vi "Main Tclk.vi"() -> ()   [LabVIEW 2018] (continued)
            n6367 = call "Email alert.vi"("Email log file path"=w2036, "Send email"=w2039, "Machine ID"=w2042, "Mail server"=w2041, "Alarm message"=w2037, "Recipents"=w2040) -> ()  [unwired: 6 in]
            n6368 = case shown="True" w2035 {
              frame False {
              }
              frame True {
                n6369 = stacked-sequence {
                  frame #0 {
                    n6370 = Wait (ms)(milliseconds to wait=u32 500) -> ()  [unwired: 1 out]
                  }
                  frame #1 {
                    w2067 = FALSE ("3D image paused active bypass")
                    n6371 = local write "Send reheat start email"(w2067) -> ()
                    "Reheat warning armed" <- w2067
                  }
                }
              }
            }
          }
          frame #14 {
            n6372 = local read "Start Reheat"() -> (w2079:bool)
            n6373 = local read "Reheat warning armed"() -> (w2078:bool)
            n6374 = local read "Reheat completed"() -> (w2075:bool)
            n6375 = local read "Machine Type"() -> (w2068:u8)
            n6376 = case shown="2" w2068 {
              tunnel: [w2098 w2120] -> w2072
              tunnel: [w2092 w2117] -> w2069
              frame 0, Default {
                w2084 = "%5.1f" ("format string")
                w2086 = "%#g" ("format string")
                n6377 = local read "Reheat Output"() -> (w2106:T21)
                n6378 = local read "HV Data Output"() -> (w2093:T18)
                n6379 = Unbundle By Name(w2106) -> ("Initial emission (uA)"=w2105:sgl, "Initial suppressor (V)"=w2104:sgl, "V/I Slope"=w2097:sgl, "Reheat Success"=w2092:bool)
                n6380 = Unbundle By Name(w2093) -> ("Suppressor (V)"=w2091:sgl, "Emission (uA)"=w2089:sgl)
                n6381 = Format Into String(format string=w2084, w2105) -> (resulting string=w2102:string)  [unwired: 2 in, 1 out]
                n6382 = Format Into String(format string=w2084, w2097) -> (resulting string=w2096:string)  [unwired: 2 in, 1 out]
                n6383 = Format Into String(format string=w2086, w2091) -> (resulting string=w2090:string)  [unwired: 2 in, 1 out]
                n6384 = Format Into String(format string=w2086, w2104) -> (resulting string=w2100:string)  [unwired: 2 in, 1 out]
                n6385 = Format Into String(format string="%3.1f", w2089) -> (resulting string=w2088:string)  [unwired: 2 in, 1 out]
                n6386 = Concatenate Strings("FIB reheat completed successfully, initial emission: " ("Alarm message"), w2102, " uA @ suppressor = " ("element"), w2100, " V, V/I slope = " ("element"), w2096, ", suppressor = " ("string"), w2090, " V @ " ("string"), w2088, " uA emission " ("string")) -> (w2098:string)
              }
              frame 2 {
                w2107 = "%3.1f" ("format string")
                n6387 = local read "Capella HV Data Output"() -> (w2118:T17)
                n6388 = local read "Reheat Output"() -> (w2121:T21)
                n6389 = Unbundle By Name(w2121) -> ("Reheat Success"=w2117:bool)
                n6390 = Unbundle By Name(w2118) -> ("Suppressor (V)"=w2116:sgl, "Emission Actual (uA)"=w2114:sgl)
                n6391 = local read "FIB V/I slope"() -> (w2109:sgl)
                n6392 = Format Into String(format string=w2107, w2109) -> (resulting string=w2108:string)  [unwired: 2 in, 1 out]
                n6393 = Format Into String(format string="%5.1f", w2116) -> (resulting string=w2115:string)  [unwired: 2 in, 1 out]
                n6394 = Format Into String(format string=w2107, w2114) -> (resulting string=w2113:string)  [unwired: 2 in, 1 out]
                n6395 = Concatenate Strings("FIB reheat completed successfully, suppressor =  " ("Alarm message"), w2115, " V @ " ("string"), w2113, " uA emission, V/I slope =  " ("string"), w2108) -> (w2120:string)
              }
            }
            n6396 = local read "Mail server"() -> (w2081:string)
            n6397 = local read "Hardware Configuration"() -> (w2083:T25)
            n6398 = Not(x=w2079) -> (.not. x?=w2076:bool)
            n6399 = Not(x=w2078) -> (.not. x?=w2077:bool)
            n6400 = Unbundle By Name(w2083) -> ("Machine ID"=w2082:string)
            n6401 = Compound Arithmetic op=AND(w2076, w2077, w2075) -> (w2080:bool)
            n6402 = local read "Email Alert Recipients"() -> (w2071:string[])
            n6403 = local read "Email Log Files"() -> (w2070:path)
            n6404 = case shown="True" w2076 {
              frame False {
              }
              frame True {
                n6405 = stacked-sequence {
                  frame #0 {
                    n6406 = Wait (ms)(milliseconds to wait=u32 500) -> ()  [unwired: 1 out]
                  }
                  frame #1 {
                    n6407 = local write "Reheat warning armed"(TRUE ("3D image paused active bypass")) -> ()
                  }
                }
              }
            }
            n6408 = Select(t=w2072, s=w2069, f="FIB reheat failed" ("Alarm message")) -> (s? t:f=w2074:string)
            n6409 = call "Email alert.vi"("Email log file path"=w2070, "Send email"=w2080, "Machine ID"=w2082, "Mail server"=w2081, "Alarm message"=w2074, "Recipents"=w2071) -> ()  [unwired: 6 in]
          }
          frame #15 {
            n6410 = local read "Email Alert Recipients"() -> (w2129:string[])
            n6411 = local read "Auto re-engage"() -> (w2125:bool)
            n6412 = local read "Re-engage warning armed"() -> (w2126:bool)
            n6413 = local read "Mail server"() -> (w2130:string)
            n6414 = local read "Hardware Configuration"() -> (w2132:T25)
            n6415 = local read "Email Log Files"() -> (w2124:path)
            n6416 = Unbundle By Name(w2132) -> ("Machine ID"=w2131:string)
            n6417 = Compound Arithmetic op=AND(w2125, w2126) -> (w2127:bool)
            n6418 = call "Email alert.vi"("Email log file path"=w2124, "Send email"=w2127, "Machine ID"=w2131, "Mail server"=w2130, "Alarm message"="Auto re-engaging started", "Recipents"=w2129) -> ()  [unwired: 6 in]
            n6419 = case shown="True" w2125 {
              frame False {
              }
              frame True {
                n6420 = stacked-sequence {
                  frame #0 {
                    n6421 = Wait (ms)(milliseconds to wait=u32 500) -> ()  [unwired: 1 out]
                  }
                  frame #1 {
                    "Re-engage warning armed" <- FALSE ("3D image paused active bypass")
                  }
                }
              }
            }
          }
          frame #16 {
            n6422 = local read "Email Alert Recipients"() -> (w2148:string[])
            n6423 = local read "Auto re-engage"() -> (w2140:bool)
            n6424 = local read "Re-engage warning armed"() -> (w2144:bool)
            n6425 = local read "Re-engage cancelled"() -> (w2136:bool)
            n6426 = local read "Re-engage counts"() -> (w2138:u8)
            n6427 = local read "Mail server"() -> (w2149:string)
            n6428 = local read "Hardware Configuration"() -> (w2151:T25)
            n6429 = local read "Email Log Files"() -> (w2141:path)
            n6430 = Not Equal?(x=w2139, y=w2138) -> (x != y?=w2137:bool)
            n6431 = Equal?(x=w2138, y=u8 50) -> (x = y?=w2142:bool)
            n6432 = Unbundle By Name(w2151) -> ("Machine ID"=w2150:string)
            n6433 = Not(x=w2144) -> (.not. x?=w2145:bool)
            n6434 = Not(x=w2136) -> (.not. x?=w2135:bool)
            n6435 = Compound Arithmetic op=AND(w2140, w2145, w2135, w2137, w2142) -> (w2146:bool)
            n6436 = call "Email alert.vi"("Email log file path"=w2141, "Send email"=w2146, "Machine ID"=w2150, "Mail server"=w2149, "Alarm message"="FI has not covered after 50 frames", "Recipents"=w2148) -> ()  [unwired: 6 in]
            n6437 = case shown="True" w2140 {
              frame False {
              }
              frame True {
                n6438 = stacked-sequence {
                  frame #0 {
                    n6439 = Wait (ms)(milliseconds to wait=u32 500) -> ()  [unwired: 1 out]
                  }
                  frame #1 {
                  }
                }
              }
            }
          }
          frame #17 {
            n6440 = local read "Email Alert Recipients"() -> (w2166:string[])
            n6441 = local read "Auto re-engage"() -> (w2158:bool)
            n6442 = local read "Re-engage warning armed"() -> (w2162:bool)
            n6443 = local read "Re-engage cancelled"() -> (w2154:bool)
            n6444 = local read "Re-engage counts"() -> (w2157:u8)
            n6445 = local read "Mail server"() -> (w2167:string)
            n6446 = local read "Hardware Configuration"() -> (w2169:T25)
            n6447 = local read "Email Log Files"() -> (w2159:path)
            n6448 = Not Equal?(x=w2156, y=w2157) -> (x != y?=w2155:bool)
            n6449 = Equal?(x=w2157, y=u8 100) -> (x = y?=w2160:bool)
            n6450 = Unbundle By Name(w2169) -> ("Machine ID"=w2168:string)
            n6451 = Not(x=w2162) -> (.not. x?=w2163:bool)
            n6452 = Not(x=w2154) -> (.not. x?=w2153:bool)
            n6453 = Compound Arithmetic op=AND(w2158, w2163, w2153, w2155, w2160) -> (w2164:bool)
            n6454 = call "Email alert.vi"("Email log file path"=w2159, "Send email"=w2164, "Machine ID"=w2168, "Mail server"=w2167, "Alarm message"="FI has not covered after 100 frames", "Recipents"=w2166) -> ()  [unwired: 6 in]
            n6455 = case shown="True" w2158 {
              frame False {
              }
              frame True {
                n6456 = stacked-sequence {
                  frame #0 {
                    n6457 = Wait (ms)(milliseconds to wait=u32 500) -> ()  [unwired: 1 out]
                  }
                  frame #1 {
                  }
                }
              }
            }
          }
          frame #18 {
            n6458 = local read "Email Alert Recipients"() -> (w2184:string[])
            n6459 = local read "Auto re-engage"() -> (w2176:bool)
            n6460 = local read "Re-engage warning armed"() -> (w2180:bool)
            n6461 = local read "Re-engage cancelled"() -> (w2172:bool)
            n6462 = local read "Re-engage counts"() -> (w2175:u8)
            n6463 = local read "Mail server"() -> (w2185:string)
            n6464 = local read "Hardware Configuration"() -> (w2187:T25)
            n6465 = local read "Email Log Files"() -> (w2177:path)
            n6466 = Not Equal?(x=w2174, y=w2175) -> (x != y?=w2173:bool)
            n6467 = Equal?(x=w2175, y=u8 200) -> (x = y?=w2178:bool)
            n6468 = Unbundle By Name(w2187) -> ("Machine ID"=w2186:string)
            n6469 = Not(x=w2180) -> (.not. x?=w2181:bool)
            n6470 = Not(x=w2172) -> (.not. x?=w2171:bool)
            n6471 = Compound Arithmetic op=AND(w2176, w2181, w2171, w2173, w2178) -> (w2182:bool)
            n6472 = call "Email alert.vi"("Email log file path"=w2177, "Send email"=w2182, "Machine ID"=w2186, "Mail server"=w2185, "Alarm message"="FI has not covered after 200 frames", "Recipents"=w2184) -> ()  [unwired: 6 in]
            n6473 = case shown="True" w2176 {
              frame False {
              }
              frame True {
                n6474 = stacked-sequence {
                  frame #0 {
                    n6475 = Wait (ms)(milliseconds to wait=u32 500) -> ()  [unwired: 1 out]
                  }
                  frame #1 {
                  }
                }
              }
            }
          }
          frame #19 {
            n6476 = local read "Auto re-engage"() -> (w2202:bool)
            n6477 = local read "Re-engage warning armed"() -> (w2200:bool)
            n6478 = local read "Re-engage cancelled"() -> (w2190:bool)
            n6479 = local read "Email Alert Recipients"() -> (w2204:string[])
            n6480 = local read "Re-engage counts"() -> (w2194:u8)
            n6481 = local read "Mail server"() -> (w2205:string)
            n6482 = local read "Hardware Configuration"() -> (w2207:T25)
            n6483 = local read "Email Log Files"() -> (w2199:path)
            n6484 = Not(x=w2202) -> (.not. x?=w2201:bool)
            n6485 = Subtract(x=w2194, y=u8 12) -> (x-y=w2193:u8)
            n6486 = Unbundle By Name(w2207) -> ("Machine ID"=w2206:string)
            n6487 = Not(x=w2200) -> (.not. x?=w2191:bool)
            n6488 = Not(x=w2190) -> (.not. x?=w2189:bool)
            n6489 = Format Into String(w2193) -> (resulting string=w2196:string)  [unwired: 3 in, 1 out]
            n6490 = Compound Arithmetic op=AND(w2201, w2191, w2189) -> (w2203:bool)
            n6491 = Concatenate Strings("Auto re-engaging finished, FI recovered in " ("Alarm message"), w2196, " frames" ("Alarm message")) -> (w2197:string)
            n6492 = call "Email alert.vi"("Email log file path"=w2199, "Send email"=w2203, "Machine ID"=w2206, "Mail server"=w2205, "Alarm message"=w2197, "Recipents"=w2204) -> ()  [unwired: 6 in]
            n6493 = case shown="True" w2201 {
              frame False {
              }
              frame True {
                n6494 = stacked-sequence {
                  frame #0 {
                    n6495 = Wait (ms)(milliseconds to wait=u32 500) -> ()  [unwired: 1 out]
                  }
                  frame #1 {
                    n6496 = local write "Re-engage warning armed"(TRUE ("3D image paused active bypass")) -> ()
                  }
                }
              }
            }
          }
          frame #20 {
            n6497 = local read "Auto re-engage"() -> (w2218:bool)
            n6498 = local read "Re-engage cancelled"() -> (w2210:bool)
            n6499 = local read "Email Alert Recipients"() -> (w2220:string[])
            n6500 = local read "Re-engage counts"() -> (w2211:u8)
            n6501 = local read "Mail server"() -> (w2221:string)
            n6502 = local read "Hardware Configuration"() -> (w2223:T25)
            n6503 = local read "Email Log Files"() -> (w2216:path)
            n6504 = Not(x=w2218) -> (.not. x?=w2217:bool)
            n6505 = Unbundle By Name(w2223) -> ("Machine ID"=w2222:string)
            n6506 = Format Into String(w2211) -> (resulting string=w2213:string)  [unwired: 3 in, 1 out]
            n6507 = Compound Arithmetic op=AND(w2217, w2210) -> (w2219:bool)
            n6508 = Concatenate Strings("Auto re-engaging cancelled after " ("Alarm message"), w2213, " frames" ("Alarm message")) -> (w2214:string)
            n6509 = call "Email alert.vi"("Email log file path"=w2216, "Send email"=w2219, "Machine ID"=w2222, "Mail server"=w2221, "Alarm message"=w2214, "Recipents"=w2220) -> ()  [unwired: 6 in]
            n6510 = case shown="True" w2217 {
              frame False {
              }
              frame True {
                n6511 = stacked-sequence {
                  frame #0 {
                    n6512 = Wait (ms)(milliseconds to wait=u32 500) -> ()  [unwired: 1 out]
                  }
                  frame #1 {
                    "Re-engage cancelled" <- FALSE ("3D image paused active bypass")
                  }
                }
              }
            }
          }
          frame #21 {
            w2227 = "%5.3f" ("format string")
            n6513 = local read "FIB"() -> (w2226:bool)
            n6514 = local read "Focus index warning active"() -> (w2231:bool)
            n6515 = local read "Alert Settings"() -> (w2235:T36)
            n6516 = local read "Email Alert Recipients"() -> (w2243:string[])
            n6517 = local read "Focus Index"() -> (w2228:sgl)
            n6518 = local read "Mail server"() -> (w2244:string)
            n6519 = local read "Hardware Configuration"() -> (w2246:T25)
            n6520 = local read "Focus index warning armed"() -> (w2241:bool)
            n6521 = Unbundle By Name(w2235) -> ("Focus index warning"=w2232:bool, "Focus index low limit"=w2234:sgl, "Run Auto Stig"=w2233:bool)
            n6522 = Unbundle By Name(w2246) -> ("Machine ID"=w2245:string)
            n6523 = Format Into String(format string=w2227, w2234) -> (resulting string=w2237:string)  [unwired: 2 in, 1 out]
            n6524 = Compound Arithmetic op=AND(w2226, w2231, w2241, w2232) -> (w2242:bool)
            n6525 = Format Into String(format string=w2227, w2228) -> (resulting string=w2240:string)  [unwired: 2 in, 1 out]
            n6526 = local read "Email Log Files"() -> (w2229:path)
            n6527 = Compound Arithmetic op=AND(w2231, w2232, w2233) -> (w2230:bool)
            n6528 = Concatenate Strings("Focus index dropped below " ("Alarm message"), w2237, " to " ("Alarm message"), w2240) -> (w2239:string)
            n6529 = call "Email alert.vi"("Email log file path"=w2229, "Send email"=w2242, "Machine ID"=w2245, "Mail server"=w2244, "Alarm message"=w2239, "Recipents"=w2243) -> ()  [unwired: 6 in]
            n6530 = case shown="True" w2231 {
              frame False {
              }
              frame True {
                n6531 = stacked-sequence {
                  frame #0 {
                    n6532 = Wait (ms)(milliseconds to wait=u32 500) -> ()  [unwired: 1 out]
                  }
                  frame #1 {
                    "Focus index warning armed" <- FALSE ("3D image paused active bypass")
                  }
                }
              }
            }
            n6533 = case shown="True" w2230 {
              frame False {
              }
              frame True {
                n6534 = local write "Auto Stig"(TRUE ("Auto Stig")) -> ()
              }
            }
          }
          frame #22 {
            w2254 = "%5.3f" ("format string")
            n6535 = local read "Focus index stop trigger active"() -> (w2259:bool)
            n6536 = local read "Alert Settings"() -> (w2262:T36)
            n6537 = local read "Email Alert Recipients"() -> (w2268:string[])
            n6538 = local read "Focus Index"() -> (w2255:sgl)
            n6539 = local read "Z removal stop threshold Z(nm)"() -> (w2250:u8)
            n6540 = local read "Mail server"() -> (w2269:string)
            n6541 = local read "Hardware Configuration"() -> (w2271:T25)
            n6542 = Unbundle By Name(w2262) -> ("Focus index warning"=w2260:bool, "Focus index stop limit"=w2261:sgl)
            n6543 = Unbundle By Name(w2271) -> ("Machine ID"=w2270:string)
            n6544 = Format Into String(format string=w2254, w2261) -> (resulting string=w2264:string)  [unwired: 2 in, 1 out]
            n6545 = Format Into String(format string=w2254, w2255) -> (resulting string=w2267:string)  [unwired: 2 in, 1 out]
            n6546 = Format Into String(format string="%d", w2250) -> (resulting string=w2252:string)  [unwired: 2 in, 1 out]
            n6547 = Compound Arithmetic op=AND(w2259, w2260) -> (w2256:bool)
            n6548 = local read "Email Log Files"() -> (w2258:path)
            n6549 = Concatenate Strings("Focus index dropped below " ("Alarm message"), w2264, " to " ("Alarm message"), w2267, " for " ("string"), w2252, "nm removal" ("string")) -> (w2266:string)
            n6550 = call "Email alert.vi"("Email log file path"=w2258, "Send email"=w2256, "Machine ID"=w2270, "Mail server"=w2269, "Alarm message"=w2266, "Recipents"=w2268) -> ()  [unwired: 6 in]
            n6551 = case shown="True" w2256 {
              frame False {
              }
              frame True {
                n6552 = stacked-sequence {
                  frame #0 {
                    n6553 = Wait (ms)(milliseconds to wait=u32 500) -> ()  [unwired: 1 out]
                  }
                  frame #1 {
                    n6554 = local write "Focus index stop trigger active"(FALSE ("Focus index stop trigger active")) -> ()
                    n6555 = local write "FI below limit counts"(u8 0 ("FI below limit counts")) -> ()
                  }
                }
              }
            }
          }
          frame #23 {
            n6556 = local read "Email Alert Recipients"() -> (w2287:string[])
            n6557 = local read "Focus index recovery active"() -> (w2284:bool)
            n6558 = local read "Focus index warning armed"() -> (w2285:bool)
            n6559 = local read "Alert Settings"() -> (w2279:T36)
            n6560 = local read "Focus Index"() -> (w2276:sgl)
            n6561 = local read "Mail server"() -> (w2288:string)
            n6562 = local read "Hardware Configuration"() -> (w2290:T25)
            n6563 = Unbundle By Name(w2279) -> ("Focus index warning"=w2278:bool)
            n6564 = Not(x=w2285) -> (.not. x?=w2280:bool)
            n6565 = Unbundle By Name(w2290) -> ("Machine ID"=w2289:string)
            n6566 = Compound Arithmetic op=AND(w2284, w2280, w2278) -> (w2286:bool)
            n6567 = Format Into String(format string="%5.3f", w2276) -> (resulting string=w2283:string)  [unwired: 2 in, 1 out]
            n6568 = local read "Email Log Files"() -> (w2277:path)
            n6569 = Concatenate Strings("Focus index recovered to " ("Alarm message"), w2283) -> (w2282:string)
            n6570 = call "Email alert.vi"("Email log file path"=w2277, "Send email"=w2286, "Machine ID"=w2289, "Mail server"=w2288, "Alarm message"=w2282, "Recipents"=w2287) -> ()  [unwired: 6 in]
            n6571 = case shown="True" w2284 {
              frame False {
              }
              frame True {
                n6572 = stacked-sequence {
                  frame #0 {
                    n6573 = Wait (ms)(milliseconds to wait=u32 500) -> ()  [unwired: 1 out]
                  }
                  frame #1 {
                    n6574 = local write "Focus index warning armed"(TRUE ("Focus index warning armed")) -> ()
                  }
                }
              }
            }
          }
          frame #24 {
            w2294 = "%5.3f" ("format string")
            n6575 = local read "Temp (F)"() -> (w2305:sgl)
            n6576 = local read "Temp range (F)"() -> (w2300:sgl)
            n6577 = local read "Temp gradient (F/min)"() -> (w2304:dbl)
            n6578 = local read "Mail server"() -> (w2313:string)
            n6579 = local read "Hardware Configuration"() -> (w2315:T25)
            n6580 = local read "Alert Settings"() -> (w2297:T36)
            n6581 = Format Into String(format string=w2294, w2305) -> (resulting string=w2309:string)  [unwired: 2 in, 1 out]
            n6582 = Format Into String(format string=w2294, w2300) -> (resulting string=w2298:string)  [unwired: 2 in, 1 out]
            n6583 = local read "Email Alert Recipients"() -> (w2312:string[])
            n6584 = local read "FIB"() -> (w2293:bool)
            n6585 = local read "Temperature warning active"() -> (w2303:bool)
            n6586 = local read "Temperature warning armed"() -> (w2302:bool)
            n6587 = Unbundle By Name(w2315) -> ("Machine ID"=w2314:string)
            n6588 = Format Into String(format string=w2294, w2304) -> (resulting string=w2307:string)  [unwired: 2 in, 1 out]
            n6589 = Unbundle By Name(w2297) -> ("Temperature alarm"=w2296:bool)
            n6590 = Concatenate Strings("Temperature reached " ("Alarm message"), w2309, " F, range @ " ("Alarm message"), w2298, " F, gradient @ " ("Alarm message"), w2307, " F/min" ("string")) -> (w2310:string)
            n6591 = local read "Email Log Files"() -> (w2295:path)
            n6592 = Compound Arithmetic op=AND(w2293, w2303, w2302, w2296) -> (w2301:bool)
            n6593 = call "Email alert.vi"("Email log file path"=w2295, "Send email"=w2301, "Machine ID"=w2314, "Mail server"=w2313, "Alarm message"=w2310, "Recipents"=w2312) -> ()  [unwired: 6 in]
            n6594 = case shown="True" w2303 {
              frame False {
              }
              frame True {
                n6595 = stacked-sequence {
                  frame #0 {
                    n6596 = Wait (ms)(milliseconds to wait=u32 500) -> ()  [unwired: 1 out]
                  }
                  frame #1 {
                    "Temperature warning armed" <- FALSE ("3D image paused active bypass")
                  }
                }
              }
            }
          }
          frame #25 {
            w2319 = "%5.3f" ("format string")
            n6597 = local read "Temp (F)"() -> (w2329:sgl)
            n6598 = local read "Temp range (F)"() -> (w2326:sgl)
            n6599 = local read "Temp gradient (F/min)"() -> (w2328:dbl)
            n6600 = local read "Mail server"() -> (w2337:string)
            n6601 = local read "Hardware Configuration"() -> (w2339:T25)
            n6602 = local read "Email Alert Recipients"() -> (w2336:string[])
            n6603 = local read "Alert Settings"() -> (w2322:T36)
            n6604 = Format Into String(format string=w2319, w2329) -> (resulting string=w2333:string)  [unwired: 2 in, 1 out]
            n6605 = Format Into String(format string=w2319, w2326) -> (resulting string=w2324:string)  [unwired: 2 in, 1 out]
            n6606 = local read "FIB"() -> (w2318:bool)
            n6607 = local read "Temperature recovery active"() -> (w2323:bool)
            n6608 = local read "Temperature warning armed"() -> (w2340:bool)
            n6609 = Format Into String(format string=w2319, w2328) -> (resulting string=w2331:string)  [unwired: 2 in, 1 out]
            n6610 = Unbundle By Name(w2322) -> ("Temperature alarm"=w2321:bool)
            n6611 = Unbundle By Name(w2339) -> ("Machine ID"=w2338:string)
            n6612 = Concatenate Strings("Temperature recovered to " ("Alarm message"), w2333, " F, range @ " ("Alarm message"), w2324, " F, gradient @ " ("Alarm message"), w2331, " F/min" ("string")) -> (w2334:string)
            n6613 = Not(x=w2340) -> (.not. x?=w2341:bool)
            n6614 = local read "Email Log Files"() -> (w2320:path)
            n6615 = Compound Arithmetic op=AND(w2318, w2323, w2341, w2321) -> (w2327:bool)
            n6616 = call "Email alert.vi"("Email log file path"=w2320, "Send email"=w2327, "Machine ID"=w2338, "Mail server"=w2337, "Alarm message"=w2334, "Recipents"=w2336) -> ()  [unwired: 6 in]
            n6617 = case shown="True" w2323 {
              frame False {
              }
              frame True {
                n6618 = stacked-sequence {
                  frame #0 {
                    n6619 = Wait (ms)(milliseconds to wait=u32 500) -> ()  [unwired: 1 out]
                  }
                  frame #1 {
                    n6620 = local write "Temperature warning armed"(TRUE ("Focus index warning armed")) -> ()
                  }
                }
              }
            }
          }
        }
        n6621 = Wait Until Next ms Multiple(millisecond multiple=u32 1000) -> ()  [unwired: 1 out]
        n6622 = local read "Stop"() -> (w1831:bool)
      }
      n6623 = Unregister For Events(event registration refnum=w713, error in=w714) -> (error out=w711:errorcluster)
      n6624 = Close Reference(reference=w715, error in (no error)=w711) -> ()  [unwired: 1 out]
      n6625 = while {
        stop <- w1208 stop-if-true
        n6626 = Wait Until Next ms Multiple(millisecond multiple=u32 100) -> ()  [unwired: 1 out]
        n6627 = case shown="True" "Load recipe" {
          frame False {
          }
          frame True {
            n6628 = stacked-sequence {
              frame #0 {
                n6629 = call "Recipe read write.vi"("Write"=FALSE, "Recipe path"="Read recipe path") -> ("Read output"=w1211:T114)  [unwired: 6 in, 3 out]
                n6630 = local read "Milling para"() -> (w1225:T35)
                n6631 = local read "FIB"() -> (w1236:bool)
                n6632 = Unbundle By Name(w1211) -> ("SEM Scan Parameters"=w1226:T5, "Detector Information"=w1227:T8, "SEM Options"=w1228:T27, "Focus Index Options"=w1210:T28, "Image fit to"=w1215:u8, "File Information"=w1229:T31, "Low mag SEM"=w1230:T30, "Mid Mag SEM"=w1219:T115, "FIB-SEM Angle"=w1231:dbl, "Milling para"=w1232:T35, "FI Detector"=w1237:u16, "Auto Optimzation"=w1238:bool, "Images per Auto Optimization"=w1239:u16, "AF Range (nm)"=w1240:sgl, "AF Steps"=w1241:u8, "AS Range (%)"=w1242:sgl, "AS Steps"=w1243:u8, "AA Range (%)"=w1217:sgl, "AA Steps"=w1216:u8, "X shift (nm/frame)"=w1234:dbl, "Y shift (nm/frame)"=w1233:dbl, "FIB Y zoom pixel (nm)"=w1235:dbl, "Mail server"=w1244:string, "Email Alert Recipients"=w1245:string[], "Alert Settings"=w1218:T116, "Reheat Parameters"=w1214:T1, "Start FIB HV DataLog"=w1213:bool, "Interval (s)"=w1212:u16)
                n6633 = local write "Recipe input"(w1211) -> ()
                n6634 = Not(x=w1236) -> (.not. x?=w1223:bool)
                n6635 = Unbundle By Name(w1225) -> ("Mill start from Last"=w1224:bool)
                n6636 = local write "Focus Index Options"(w1210) -> ()
                n6637 = local write "Image fit to"(w1215) -> ()
                n6638 = local write "FI Detector"(w1237) -> ()
                n6639 = local write "Auto Optimzation"(w1238) -> ()
                n6640 = local write "Images per Auto Optimization"(w1239) -> ()
                n6641 = local write "AF Range (nm)"(w1240) -> ()
                n6642 = local write "AF Steps"(w1241) -> ()
                n6643 = local write "AS Range (%)"(w1242) -> ()
                n6644 = local write "AS Steps"(w1243) -> ()
                n6645 = local write "AA Range (%)"(w1217) -> ()
                n6646 = local write "AA Steps"(w1216) -> ()
                n6647 = local write "Alert Settings"(w1218) -> ()
                n6648 = local write "Reheat Parameters"(w1214) -> ()
                n6649 = local write "Start FIB HV DataLog"(w1213) -> ()
                n6650 = local write "Interval (s)"(w1212) -> ()
                n6651 = Or(x=w1224, y=w1223) -> (x .or. y?=w1222:bool)
                n6652 = case shown="True" w1222 {
                  tunnel: w1226 -> [w1249 w1306]
                  tunnel: w1227 -> [_ w1292]
                  tunnel: w1228 -> [_ w1305]
                  tunnel: w1229 -> [_ w1304]
                  tunnel: w1230 -> [w1248 w1303]
                  tunnel: w1231 -> [_ w1302]
                  tunnel: w1232 -> [w1247 w1301]
                  tunnel: w1233 -> [_ w1300]
                  tunnel: w1234 -> [_ w1299]
                  tunnel: w1235 -> [_ w1298]
                  tunnel: w1244 -> [_ w1297]
                  tunnel: w1245 -> [_ w1296]
                  tunnel: w1219 -> [w1246 w1295]
                  frame False {
                    n6653 = stacked-sequence {
                      tunnel: w1249 -> [w1260 _ _]
                      tunnel: w1248 -> [_ w1280 _]
                      tunnel: w1247 -> [_ _ w1286]
                      tunnel: w1246 -> [_ w1272 _]
                      frame #0 {
                        n6654 = Unbundle By Name(w1260) -> ("X size (um)"=w1259:sgl, "Y size (um)"=w1258:sgl, "X size (V)"=w1257:dbl, "X size auto"=w1256:bool, "Scan rate (Hz)"=w1255:u32, "Oversampling"=w1254:u32, "Oversampling auto"=w1253:bool, "Frame line rampdown ratio"=w1252:sgl, "Pixel size (nm)"=w1251:sgl)
                        n6655 = local read "SEM Scan Parameters"() -> (w1261:T26)
                        n6656 = Bundle By Name(cluster=w1261, "X size (um)"=w1259, "Y size (um)"=w1258, "X size (V)"=w1257, "X size auto"=w1256, "Scan rate (Hz)"=w1255, "Oversampling"=w1254, "Oversampling auto"=w1253, "Frame line rampdown ratio"=w1252, "Pixel size (nm)"=w1251) -> (w1250:T26)
                        n6657 = local write "SEM Scan Parameters"(w1250) -> ()
                      }
                      frame #1 {
                        n6658 = Unbundle By Name(w1280) -> ("Low mag scan"=w1277:bool, "Prior to main scan"=w1276:bool, "Low mag interval"=w1275:u32, "Low mag scan rate (Hz)"=w1274:u32, "Show HM box"=w1273:bool)
                        n6659 = Unbundle By Name(w1272) -> ("Mid mag scan"=w1269:bool, "Prior to main scan"=w1268:bool, "Mid mag interval"=w1267:u32, "X size (um)"=w1266:sgl, "Y size (um)"=w1265:sgl, "Mid mag scan rate (Hz)"=w1264:u32, "Pixel size (nm)"=w1263:dbl, "Show MM box"=w1262:bool)
                        n6660 = local read "Mid Mag SEM"() -> (w1270:T29)
                        n6661 = Bundle By Name(cluster=w1270, "Mid mag scan"=w1269, "Prior to main scan"=w1268, "Mid mag interval"=w1267, "X size (um)"=w1266, "Y size (um)"=w1265, "Mid mag scan rate (Hz)"=w1264, "Pixel size (nm)"=w1263, "Show MM box"=w1262) -> (w1271:T29)
                        n6662 = local read "Low Mag SEM"() -> (w1279:T30)
                        n6663 = Bundle By Name(cluster=w1279, "Low mag scan"=w1277, "Prior to main scan"=w1276, "Low mag interval"=w1275, "Low mag scan rate (Hz)"=w1274, "Show HM box"=w1273) -> (w1278:T30)
                        n6664 = local write "Low Mag SEM"(w1278) -> ()
                        n6665 = local write "Mid Mag SEM"(w1271) -> ()
                      }
                      frame #2 {
                        n6666 = Unbundle By Name(w1286) -> ("Line milling time (s)"=w1283:sgl, "Lines auto pause"=w1282:u16, "Auto Profile"=w1281:bool)
                        n6667 = local read "Milling para"() -> (w1285:T35)
                        n6668 = Bundle By Name(cluster=w1285, "Line milling time (s)"=w1283, "Lines auto pause"=w1282, "Auto Profile"=w1281) -> (w1284:T35)
                        n6669 = local write "Milling para"(w1284) -> ()
                      }
                    }
                  }
                  frame True {
                    n6670 = local write "SEM Scan Parameters"(w1306) -> ()
                    n6671 = local write "Detector Information"(w1292) -> ()
                    n6672 = local write "SEM Options"(w1305) -> ()
                    n6673 = local write "File Information"(w1304) -> ()
                    n6674 = local write "Low Mag SEM"(w1303) -> ()
                    n6675 = local write "Mid Mag SEM"(w1295) -> ()
                    n6676 = local write "FIB-SEM Angle"(w1302) -> ()
                    n6677 = local write "Milling para"(w1301) -> ()
                    n6678 = local write "X shift (nm/image)"(w1299) -> ()
                    n6679 = local write "Y shift (nm/image)"(w1300) -> ()
                    n6680 = local write "FIB Y zoom pixel (nm)"(w1298) -> ()
                    n6681 = local write "Mail server"(w1297) -> ()
                    n6682 = local write "Email Alert Recipients"(w1296) -> ()
                    n6683 = Unbundle By Name(w1292) -> ("Brightness A"=w1291:dbl, "Contrast A"=w1290:dbl, "Detector B name"=w1289:string, "Brightness B"=w1288:dbl, "Contrast B"=w1287:dbl)
                    n6684 = local read "Hardware Configuration"() -> (w1294:T25)
                    n6685 = Bundle By Name(cluster=w1294, "Brightness A"=w1291, "Contrast A"=w1290, "Detector B name"=w1289, "Brightness B"=w1288, "Contrast B"=w1287) -> (w1293:T25)
                    n6686 = local write "Hardware Configuration"(w1293) -> ()
                  }
                }
              }
              frame #1 {
                n6687 = local read "Milling para"() -> (w1329:T35)
                n6688 = local read "FIB"() -> (w1328:bool)
                n6689 = case shown="False" w1328 {
                  tunnel: [TRUE ("Origin") FALSE ("Origin")] -> w1327
                  tunnel: [0.0 ("Y offset pre (um)") w1332] -> w1309
                  frame False {
                  }
                  frame True {
                    n6690 = local read "Y offset pre (um)"() -> (w1332:dbl)
                  }
                }
                n6691 = Unbundle By Name(w1329) -> ("X size (um)"=w1316:sgl, "Z size (um)"=w1317:sgl, "Z-step (nm)"=w1307:dbl)
                n6692 = expression code="x/1e3"(w1307) -> (w1319:dbl)
                n6693 = control-ref of="FIB Image"() -> (w1323:refnum<vi>)
                n6694 = local read "FIB Scan Parameters"() -> (w1324:T32)
                n6695 = local read "FIB Options"() -> (w1325:T33)
                n6696 = shared-variable ".\\Zeiss Library.lvlib\\Milling Z Voltage RT"() -> (w1326:sgl)  [unwired: 1 in, 1 out]
                n6697 = expression code="log2( x/0.1)"(w1316) -> (w1314:sgl)
                n6698 = Round Toward +Infinity(x=w1314) -> (ceil(x): smallest int >= x=w1312:sgl)
                n6699 = call "FIB image draw milling.vi"("Milling Z Voltage"=w1326, "Milling para"=w1329, "Z offset pre (um)"=w1309, "FIB Options"=w1325, "FIB Scan Parameters"=w1324, "Origin"=w1327, "Image reference"=w1323) -> ("Trapezoidal"=w1308:cluster{"X":i16, "Y":i16}[])  [unwired: 3 in, 1 out]
                n6700 = Scale By Power Of 2(n=w1312, x=ext 1.0) -> (x*2^n=w1315:ext)
                n6701 = local write "Trapezoidal"(w1308) -> ()
                n6702 = Divide(x=w1317, y=w1319) -> (x/y=w1311:dbl)
                n6703 = Round To Nearest(number=w1311) -> (nearest integer value=w1322:dbl)
                n6704 = local read "Milling para"() -> (w1320:T35)
                n6705 = Increment(x=w1322) -> (x+1=w1321:dbl)
                n6706 = Multiply(x=w1322, y=w1319) -> (x*y=w1318:dbl)
                n6707 = Bundle By Name(cluster=w1320, "X resolution"=w1315, "Z resolution"=w1321, "Z size (um)"=w1318) -> (w1310:T35)
                n6708 = local write "Milling para"(w1310) -> ()
              }
              frame #2 {
                n6709 = local read "dat to csv and xml"() -> (w1334:bool)
                n6710 = local write "Load recipe"(FALSE ("Load recipe")) -> ()
                n6711 = case shown="True" w1334 {
                  frame False {
                  }
                  frame True {
                    n6712 = stacked-sequence {
                      frame #0 {
                        w1350 = i16 60 ("top")
                        n6713 = local read "SEM Scan Parameters"() -> (w1345:T26)
                        n6714 = local read "Recipe input"() -> (w1378:T7)
                        n6715 = local read "Last FIB recipe"() -> (w1379:path)
                        n6716 = local read "Read recipe path"() -> (w1364:path)
                        n6717 = Path To String(path=w1364) -> (string=w1363:string)
                        n6718 = call "Recipe read write.vi"("Write"=TRUE, "Recipe path"=w1379, "Write input"=w1378) -> ()  [unwired: 5 in, 4 out]
                        n6719 = call "Zeiss File Header Tclk.vi"("Write"=FALSE, "Input file path"=w1364) -> ("Ouputs"=w1373:T79)  [unwired: 7 in, 2 out]
                        n6720 = Unbundle By Name(w1345) -> ("X size (um)"=w1344:sgl, "Y size (um)"=w1341:sgl, "Pixel size (nm)"=w1343:sgl)
                        n6721 = local read "Hardware Configuration"() -> (w1337:T25)
                        n6722 = Unbundle By Name(w1373) -> ("Data Logging.Milling Z voltage (V)"=w1371:sgl, "Data Logging.FIB slice #"=w1369:u32, "Data Logging.Focus Index"=w1368:sgl, "Decimating factor"=w1338:u16)
                        n6723 = call "Timestamp from dat file.vi"("dat file path"=w1364) -> ("time stamp"=w1370:timestamp)  [unwired: 10 in]
                        n6724 = Search and Replace String(input string=w1363, search string=".dat", replace string=".png" ("replace string (\"\")")) -> (result string=w1360:string)  [unwired: 5 in, 3 out]
                        n6725 = String To Path(string=w1360) -> (path=w1359:path)
                        n6726 = local read "Last milling snapshot"() -> (w1374:path)
                        n6727 = expression code="x/1000"(w1343) -> (w1342:sgl)
                        n6728 = Divide(x=w1344, y=w1342) -> (x/y=w1340:sgl)
                        n6729 = Divide(x=w1341, y=w1342) -> (x/y=w1339:sgl)
                        n6730 = Unbundle By Name(w1337) -> ("SEM Max FOV (um)"=w1336:sgl)
                        n6731 = Divide(x=w1340, y=w1338) -> (x/y=w1352:sgl)
                        n6732 = Divide(x=w1339, y=w1338) -> (x/y=w1349:sgl)
                        n6733 = To Word Integer(number=w1352) -> (16bit integer=w1348:i16)
                        n6734 = To Word Integer(number=w1349) -> (16bit integer=w1347:i16)
                        n6735 = local read "Re-engage Files"() -> (w1354:path)
                        n6736 = Bundle(cluster=T47 {"Timestamp"=timestamp(0 s since 1904-01-01), "Double"=0.0, "FIB slice #"=0, "Reheat"=FALSE, "Double 2"=0.0, "Double 3"=0.0, "Double 4"=0.0} ("output cluster"), "Timestamp"=w1370, "Double"=w1371, "FIB slice #"=w1369, "Reheat"=TRUE, "Double 2"=w1368, "Double 3"=w1368, "Double 4"=w1336) -> (w1375:T47)
                        n6737 = call <vilib>:"Read PNG File.vi"("path to PNG file"=w1359) -> ("image data"=w1346:T55)  [unwired: 8 in, 2 out]
                        n6738 = Add(x=w1350, y=w1347) -> (x+y=w1351:i16)
                        n6739 = Flatten To XML(anything=w1375) -> (xml string=w1376:string)
                        n6740 = Bundle By Name(cluster=T46 {"left"=0, "top"=0, "right"=0, "bottom"=0} ("subset rect"), "left"=i16 0, "top"=w1350, "right"=w1348, "bottom"=w1351) -> (w1356:T46)
                        n6741 = call-poly <vilib>:"Write to XML File.vi"("XML Input"=w1376, "XML File Path"=w1374) -> ()  [unwired: 7 in, 3 out]
                        n6742 = call <vilib>:"Get Image Subset.vi"("subset rect"=w1356, "image data"=w1346) -> ("image subset"=w1365:T55)  [unwired: 4 in, 1 out]
                        n6743 = Build Path(base path=w1354, name or relative path="pre.png") -> (appended path=w1353:path)
                        n6744 = call <vilib>:"Write PNG File.vi"("image data"=w1365, "path to PNG file"=w1353) -> ()  [unwired: 1 in, 9 out]
                      }
                      frame #1 {
                        n6745 = local write "dat to csv and xml"(FALSE ("dat to csv and xml")) -> ()
                        n6746 = local read "Milling para"() -> (w1380:T35)
                        n6747 = Bundle By Name(cluster=w1380, "Mill start from Last"=TRUE) -> (w1382:T35)
                        n6748 = local write "Milling para"(w1382) -> ()
                      }
                    }
                  }
                }
              }
            }
          }
        }
        n6749 = local read "Stop"() -> (w1208:bool)
      }
      n6750 = while {
        shift-right: [w1467] -> _
        shift-left: w708 -> [w1466]
        shift-right: [w1462] -> _
        shift-left: _ -> [w1463]
        shift-right: [w1457] -> _
        shift-left: w708 -> [w1456]
        shift-right: [w1455] -> _
        shift-left: w708 -> [w1445]
        shift-right: [w1448] -> _
        shift-left: w708 -> [w1447]
        shift-right: [w1440] -> _
        shift-left: w708 -> [w1439]
        shift-right: ["Start FIB HV DataLog"] -> _
        shift-left: _ -> [w1438]
        shift-right: [w1434] -> _
        shift-left: w708 -> [w1429]
        shift-right: [w1425] -> _
        shift-left: w708 -> [w1418]
        stop <- w1464 stop-if-true
        n6751 = local read "FIB"() -> (w1450:bool)
        n6752 = local read "FIB slice #"() -> (w1444:u32)
        n6753 = local read "Mill Manual Pause"() -> (w1442:bool)
        n6754 = local read "SW error warning armed"() -> (w1426:bool)
        n6755 = local read "Alert Settings"() -> (w1405:T36)
        n6756 = local read "Milling para"() -> (w1403:T35)
        n6757 = Tick Count (ms)() -> (millisecond timer value=w1462:u32)
        n6758 = Equal To 0?(x=w1445) -> (x = 0?=w1451:bool)
        n6759 = local read "Machine Type"() -> (w1427:u8)
        n6760 = Equal To 0?(x=w1429) -> (x = 0?=w1428:bool)
        n6761 = Equal To 0?(x=w1418) -> (x = 0?=w1417:bool)
        n6762 = Subtract(x=w1462, y=w1463) -> (x-y=w1421:u32)
        n6763 = Not Equal?(x=w1438, y="Start FIB HV DataLog") -> (x != y?=w1437:bool)
        n6764 = Equal To 0?(x=w1456) -> (x = 0?=w1388:bool)
        n6765 = Not Equal To 0?(x=w1444) -> (x != 0?=w1443:bool)
        n6766 = And(x=w1437, y="Start FIB HV DataLog") -> (x .and. y?=w1436:bool)
        n6767 = Unbundle By Name(w1403) -> ("Lines auto pause"=w1402:u16)
        n6768 = Wait Until Next ms Multiple(millisecond multiple=u32 1000) -> ()  [unwired: 1 out]
        n6769 = Unbundle By Name(w1405) -> ("SW error warning"=w1404:bool)
        n6770 = Compound Arithmetic op=AND(w1417, "Start Current DataLog") -> (w1415:bool)
        n6771 = Not(x=w1442) -> (.not. x?=w1441:bool)
        n6772 = case shown="True" w1388 {
          frame False {
          }
          frame True {
            w1694 = 10.0 ("y")
            w1700 = 50 ("sample length")
            n6773 = local read "Hardware Configuration"() -> (w1686:T25)
            n6774 = for {
              N: w1700 -> [_]
              tunnel: [w1711] -> w1699 mode=indexing
              i -> [w1711]
            }
            n6775 = Unbundle By Name(w1686) -> ("Temperature port"=w1687:refnum<visa-resource-name>)
            n6776 = for {
              N: 3 -> [_]
              tunnel: w1687 -> [w1709]
              tunnel: [w1706] -> w1704
              stop <- w1707 stop-if-true
              w1710 = TRUE ("Close session")
              n6777 = call "Watchport Comm.vi"("Close session"=w1710, "Initialization"=w1710, "Watchport command"="TF", "Watchport COM #"=w1709) -> ("value"=w1706:sgl)  [unwired: 3 in, 4 out]
              n6778 = Not Equal To 0?(x=w1706) -> (x != 0?=w1707:bool)
              n6779 = Wait Until Next ms Multiple(millisecond multiple=u32 100) -> ()  [unwired: 1 out]
            }
            "Temp (F)" <- w1704
            n6780 = call <vilib>:"Data Queue PtByPt.vi"("sample length"=w1700, "input data point"=w1704) -> ("Current Queue"=w1701:dbl[])  [unwired: 5 in, 4 out]
            n6781 = call "Remove value from array.vi"("Value to remove"=0.0, "Input array"=w1701) -> ("Output array"=w1691:dbl[])  [unwired: 8 in, 1 out]
            n6782 = Array Size(array=w1691) -> (size(s)=w1692:i32)
            n6783 = Array Subset(array=w1699, length=w1692) -> (w1698:i32[])  [unwired: 1 in]
            n6784 = call <vilib>:"Linear Fit.vi"("Y"=w1691, "X"=w1698) -> ("slope"=w1703:dbl)  [unwired: 9 in, 4 out]
            n6785 = Multiply(x=w1703, y=w1694) -> (x*y=w1697:dbl)
            n6786 = Less Or Equal?(x=w1694, y=w1692) -> (x <= y?=w1693:bool)
            n6787 = Select(t=w1697, s=w1693, f=0.0) -> (s? t:f=→"Temp gradient (F/min)":dbl)
            n6788 = Array Max & Min(array=w1691) -> (max value=w1690:dbl, min value=w1689:dbl)  [unwired: 2 out]
            n6789 = Subtract(x=w1690, y=w1689) -> (x-y=→"Temp range (F)":dbl)
          }
        }
        n6790 = Add(x=w1421, y=w1445) -> (x+y=w1454:u32)
        n6791 = case shown="True" "Start FIB HV DataLog" {
          tunnel: [u32 0 ("f") w1536] -> w1440
          tunnel: w1421 -> [_ w1535]
          tunnel: w1439 -> [_ w1534]
          tunnel: w1436 -> [_ w1533]
          tunnel: w1427 -> [_ w1532]
          frame False {
          }
          frame True {
            n6792 = case shown="0" w1532 {
              tunnel: [w1545 u32 0 ("f") w1613] -> w1536
              tunnel: w1535 -> [w1544 _ w1612]
              tunnel: w1534 -> [w1543 _ w1611]
              tunnel: w1533 -> [w1540 _ w1607]
              frame 0 {
                n6793 = Equal To 0?(x=w1543) -> (x = 0?=w1538:bool)
                n6794 = local read "Re-read HVDataLog"() -> (w1539:bool)
                n6795 = Or(x=w1538, y=w1539) -> (x .or. y?=w1537:bool)
                n6796 = case shown="True" w1537 {
                  tunnel: w1540 -> [_ w1549]
                  frame False {
                  }
                  frame True {
                    n6797 = stacked-sequence {
                      tunnel: w1549 -> [w1550 _]
                      frame #0 {
                        n6798 = local read "FIB HV DataLog Files"() -> (w1551:path)
                        n6799 = Get Date/Time In Seconds() -> (seconds since 1Jan1904=w1558:timestamp)
                        n6800 = case shown="True" w1550 {
                          frame False {
                          }
                          frame True {
                            w1560 = 0.0
                            n6801 = Get Date/Time In Seconds() -> (seconds since 1Jan1904=w1570:timestamp)
                            n6802 = To Double Precision Float(number=w1570) -> (double precision float=w1565:dbl)
                            n6803 = Bundle(w1560, w1560) -> (w1559:cluster{dbl, dbl})  [unwired: 1 in]
                            n6804 = Add(x=w1565, y=86400.0 ("X Scale.Range:Maximum")) -> (x+y=w1567:dbl)
                            n6805 = Initialize Array(w1559, 0) -> (w1562:cluster{dbl, dbl}[])
                            n6806 = Add(x=w1565, y=0.0 ("X Scale.Range:Minimum")) -> (x+y=w1563:dbl)
                            n6807 = property on="FIB HV DataLog" class="WFChart (strict)"("History Data"=w1562, "XScale.Offset"=w1565, "XScale.Minimum"=w1563, "XScale.Maximum"=w1567, "XScale.Increment"=14400.0 ("X Scale.Range:Increment"), "XScale.MinorInc"=3600.0 ("X Scale.Range:Minor Increment")) -> ()  [unwired: 2 in, 2 out]
                          }
                        }
                        n6808 = Format Date/Time String(time format string (%c)="Y%Y\\M%m\\D%d", seconds (now)=w1558) -> (date/time string=w1554:string)  [unwired: 1 out]
